vi "2 station_keeping_circles.vi"(10 "Mission in":refnum<class "Mission.lvclass">) -> (2 "No Sail Circles":T1[](array[typedef]))   [LabVIEW 2011]
uses:
  2 Classes/Mission/Mission.lvclass
  2 Typedefs/UTM Circle.ctl
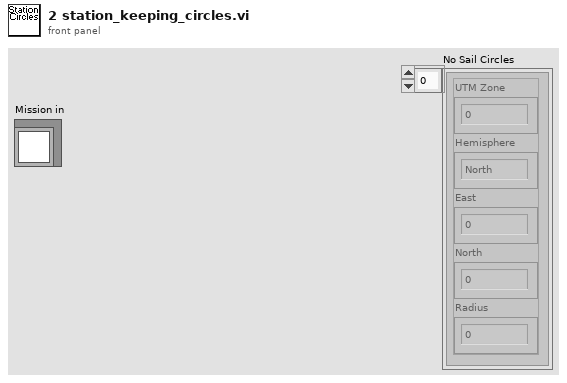
[diagram p1: front panel]
types:
  T1 = typedef "UTM Circle.ctl" = cluster{"UTM Zone":dbl, "Hemisphere":enum16{"North", "South"}, "East":dbl, "North":dbl, "Radius":dbl}
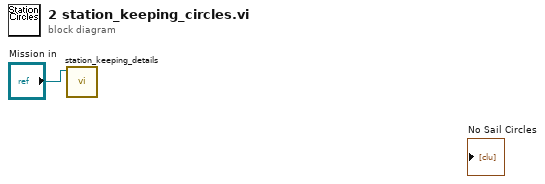
[diagram p0: block diagram]
diagram:
  n1 = call-dynamic "station_keeping_details.vi"("Mission in"="Mission in") -> ()  [unwired: 5 in, 6 out]
